vi "Get last data point.vi"(8 "error in (no error)":errorcluster, 11 "Automatic Mode in":refnum<class "Automatic Mode.lvclass">) -> (0 "error out":errorcluster, 1 "Polarization":dbl, 2 "Eventnum":i64, 3 "Automatic Mode out":refnum<class "Automatic Mode.lvclass">)   [LabVIEW 2019, in "Automatic Mode.lvclass"]
uses:
  Automatic Mode.lvclass
  Automatic Mode.lvclass/Automatic Mode.ctl
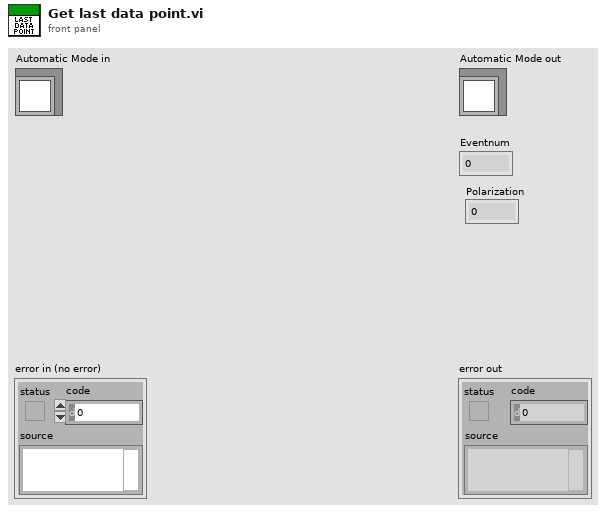
[diagram p1: front panel]
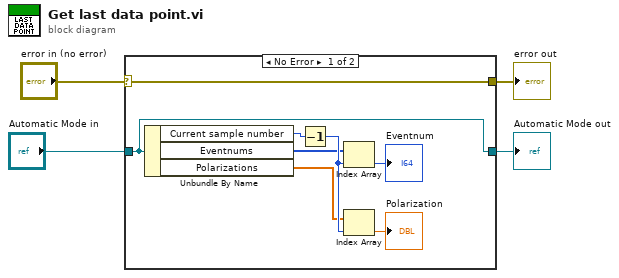
[diagram p0: block diagram]
diagram:
  n1 = case shown="No Error" "error in (no error)" {
    selector: "error in (no error)" -> [w12 w14]
    tunnel: [w12 w14] -> w3
    tunnel: [w11 w13] -> w1
    tunnel: "Automatic Mode in" -> [w11 w13]
    frame No Error {
      n2 = Unbundle By Name(w11) -> ("Current sample number"=w10:i32, "Eventnums"=w8:i64[], "Polarizations"=w6:dbl[])
      n3 = Decrement(x=w10) -> (x-1=w9:i32)
      n4 = Index Array(array=w8, index=w9) -> (element=→"Eventnum":i64)
      n5 = Index Array(array=w6, index=w9) -> (element=→"Polarization":dbl)
    }
    frame Error {
    }
  }
  "error out" <- w3
  "Automatic Mode out" <- w1
